vi "ResizeAnnulus.vi"(4 "y":dbl, 5 "Input Annulus":T2 {"End Angle" min=-90.0 max=90.0 step=1.0 format="%.2f"; "Start Angle" min=-90.0 max=90.0 step=1.0 format="%.2f"; "Center X" scale=0.0..1024.0}) -> (2 "Output Annulus":T1)   [LabVIEW 2014]
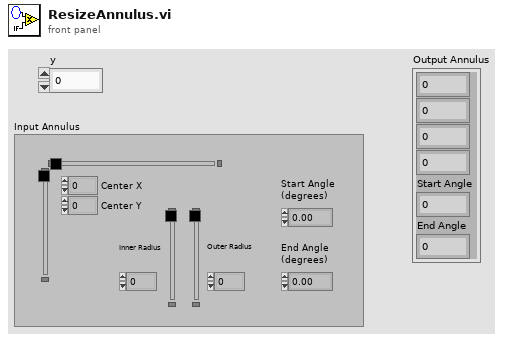
[diagram p1: front panel]
types:
  T1 = cluster{dbl, dbl, dbl, dbl, "Start Angle":dbl, "End Angle":dbl}
  T2 = typedef "IMAQ Circle" = cluster{"Center X":i32, "Center Y":i32, "Inner Radius":i32, "Outer Radius":i32, "Start Angle":dbl, "End Angle":dbl}
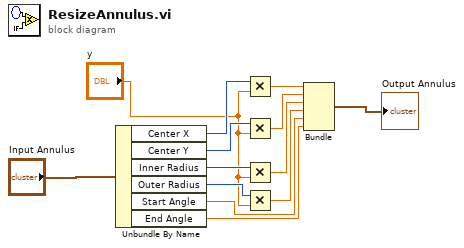
[diagram p0: block diagram]
diagram:
  n1 = Unbundle By Name("Input Annulus") -> ("Center X"=w13:i32, "Center Y"=w12:i32, "Inner Radius"=w11:i32, "Outer Radius"=w10:i32, "Start Angle"=w5:dbl, "End Angle"=w4:dbl)
  n2 = Multiply(x=w13, y="y") -> (x*y=w9:dbl)
  n3 = Multiply(x=w12, y="y") -> (x*y=w8:dbl)
  n4 = Multiply(x=w11, y="y") -> (x*y=w7:dbl)
  n5 = Multiply(x=w10, y="y") -> (x*y=w6:dbl)
  n6 = Bundle(w9, w8, w7, w6, "Start Angle"=w5, "End Angle"=w4) -> (→"Output Annulus":T1)  [unwired: 1 in]
